vi "Set-state-display.vi"(8 "error in":errorcluster, 9 "State":T1, 11 "UI ref. in":refnum<data-value>) -> (0 "error IO":errorcluster, 3 "UI ref.":refnum<data-value>)   [LabVIEW 2013, in "CameraVision.lvlib" / "CV-UI.lvclass"]
doc: "This function resets the values of the GUI buttons and selectors to consistent defaults.\nThe purpose is to present a consistent GUI after an unexpected program shutdown."
uses:
  CV-UI.lvclass
  Main/Application-states.ctl
  Display-names.ctl
  CV-UI.lvclass/CV-UI.ctl
  Read Display refs.vi
  Main/CV-Main.lvclass
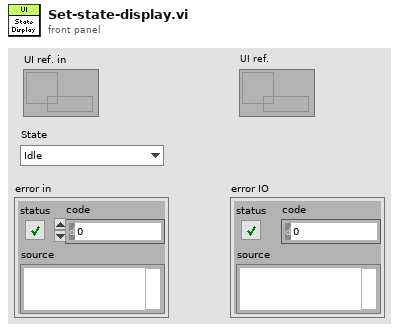
[diagram p1: front panel]
types:
  T1 = typedef "CameraVision.lvlib/CV-Main.lvclass/Application-states.ctl" = enum16{"Idle", "Initialized", "Configured", "Activated", "Started", "Stopped", "Reset", "Error", "Exited"}
  T2 = typedef "CameraVision.lvlib/CV-UI.lvclass/Display-names.ctl" = enum16{"State", "Action", "Current image", "Framerate", "Frametime", "Process buffer", "Storage buffer", "Free disk space", "Total disk space", "Information", "Histogram", "Camera 1", "Camera 2", "Camera 1 chart", "Camera 2 chart", "Browser", "Temperature", "Map", "Status overview", "Characteristics", "Temper characteristics"}
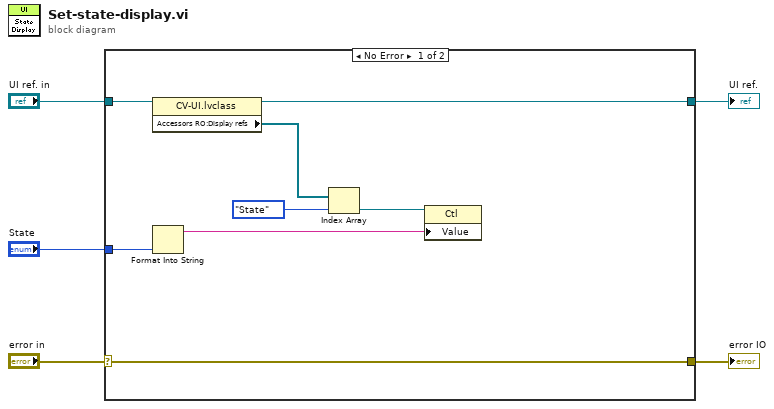
[diagram p0: block diagram]
diagram:
  n1 = case shown="No Error" "error in" {
    selector: "error in" -> [w10 w15]
    tunnel: "UI ref. in" -> [w12 w14]
    tunnel: [w10 w15] -> w5
    tunnel: [w11 w14] -> w2
    tunnel: "State" -> [w8 _]
    frame No Error {
      n2 = property class="CV-UI.lvclass"(reference=w12) -> (reference out=w11:refnum<data-value>, "Accessors RO:Display refs"=w13:refnum<vi>[])  [unwired: 1 in, 1 out]
      n3 = Format Into String(w8) -> (resulting string=w7:string)  [unwired: 3 in, 1 out]
      n4 = Index Array(array=w13, index=Display-names."State" ("Dislay")) -> (element=w9:refnum<vi>)
      n5 = property class="Ctl"(reference=w9, "Value"=w7) -> ()  [unwired: 1 in, 2 out]
    }
    frame Error {
    }
  }
  "error IO" <- w5
  "UI ref." <- w2
